vi "DtCreateCtrPeriodChan.vi"(5 "Board Name":string, 7 "Counter Num":u32, 9 "Input Line":i32(ring) items=["ClockInput", "GateInput"], 11 "error in (no error)":errorcluster) -> (4 "Task out":i32, 15 "error out":errorcluster)   [LabVIEW 2022 SP3]
doc: "Creates one or more virtual counter/timer channels that measure the period, in milliseconds, of an external digital signal that is connected to the counter/timer's clock input or gate input source."
uses:
  DtLvLink.lvlib
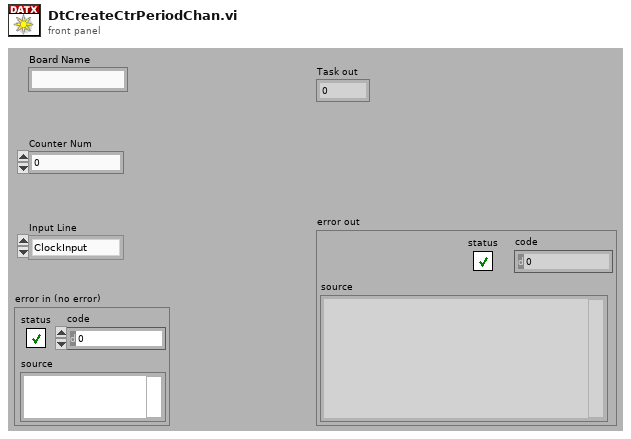
[diagram p1: front panel]
types:
  T1 = enum32{"AnalogInput", "AnalogOutput", "DigitalInput", "DigitalOutput", "Quadrature", "CounterTimer"}
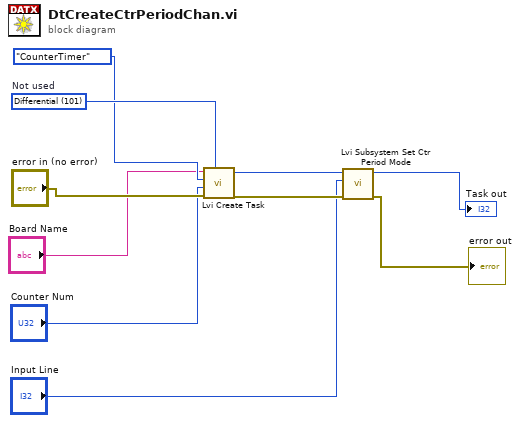
[diagram p0: block diagram]
diagram:
  w10 = 101 items=["SingleEnded"=100, "Differential"=101]  # Not used
  n1 = call "Lvi Create Task.vi"("SEorDiff"=w10, "error in (no error)"="error in (no error)", "SubSysIndex"="Counter Num", "ChanType"=T1."CounterTimer", "BoardName"="Board Name") -> ("error out"=w4:errorcluster, "TaskRef"=w5:i32)  [unwired: 4 in, 1 out]
  n2 = call "Lvi Subsystem Set Ctr Period Mode.vi"("error in (no error)"=w4, "InputLine"="Input Line", "TaskRef"=w5) -> ("error out"=→"error out":errorcluster, "TaskRef out"=→"Task out":i32)  [unwired: 6 in, 1 out]
